vi "ResolutionRingToEnum.vi"(11 "Resolution(Enum)":u32(ring)=10 items=["1000 points"=1, "10k points"=10, "100k points"=100, "1M points"=1000, "5M points"=5000, "10M points"=10000]) -> (3 "Resolution(Ring)":T1)   [LabVIEW 2013]
uses:
  shared/Typdefs/Choice77.ctl
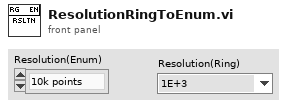
[diagram p1: front panel]
types:
  T1 = typedef "Choice77.ctl" = enum16{"1E+3", "10E+3", "100E+3", "1E+6", "5E+6", "10E+6"}
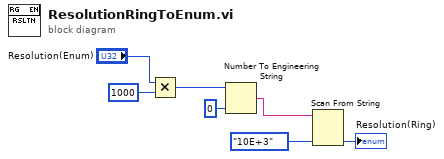
[diagram p0: block diagram]
diagram:
  n1 = Multiply(x="Resolution(Enum)", y=u32 1000) -> (x*y=w5:u32)
  n2 = Number To Engineering String(2:i16 0 ("precision (6)"), 4:w5) -> (0:w3:string)  [unwired: 2 in]
  n3 = Scan From String(input string=w3, default 1=Choice77."10E+3" ("resolution")) -> (output 1=→"Resolution(Ring)":T1)  [unwired: 3 in, 3 out]
